vi "FTW-Messenger-AsynchronousInitRequest.vi"(0 "Messenger Type":refnum<class "FTW-Messenger.lvclass">, 11 "error in":errorcluster) -> (4 "Messenger":refnum<class "FTW-Messenger.lvclass">, 15 "error out":errorcluster)   [LabVIEW 2013, in "FTW-Messenger.lvclass"]
uses:
  FTW-Messenger.lvclass
  Container/FTW-Container.lvclass
  FTW-Messenger.lvclass/FTW-Messenger.ctl
panel:
  # "Inputs"
  # "Outputs"
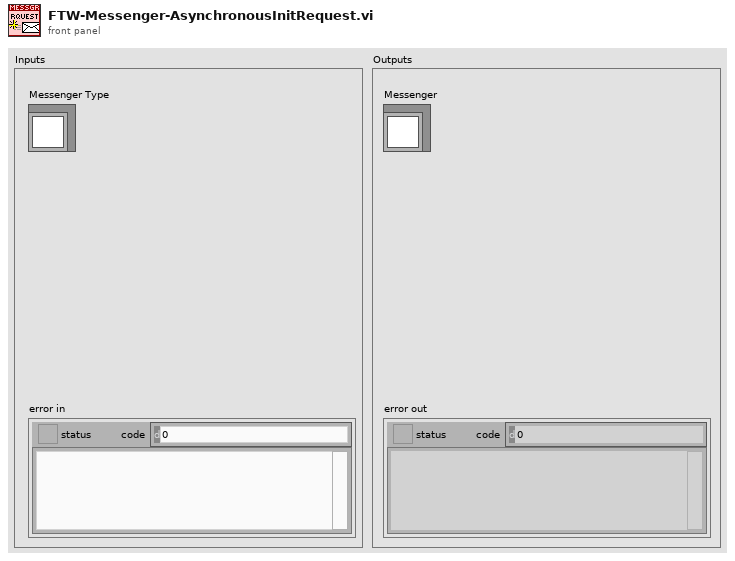
[diagram p1: front panel]
types:
  T1 = cluster{"Response":refnum<class "FTW-Container.lvclass">, "Messenger":refnum<class>}
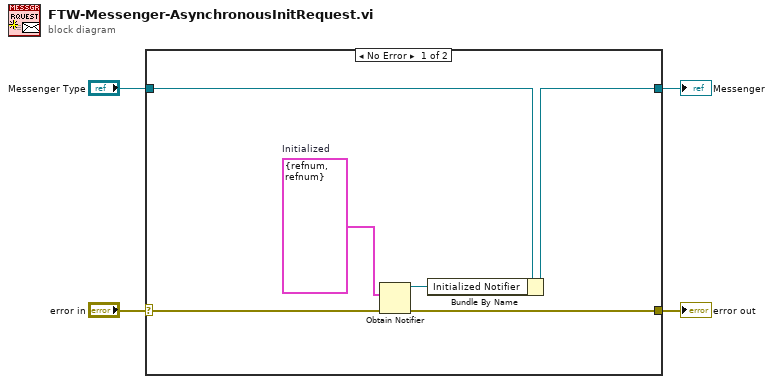
[diagram p0: block diagram]
diagram:
  n1 = case shown="No Error" "error in" {
    selector: "error in" -> [w10 w12]
    tunnel: [w8 w12] -> w3
    tunnel: [w9 w11] -> w4
    tunnel: "Messenger Type" -> [w7 w11]
    frame No Error {
      w5 = T1 {"Response"=refnum, "Messenger"=refnum}  # Initialized
      n2 = Obtain Notifier(notification data type=w5, error in (no error)=w10) -> (notifier out=w6:refnum<notifier>, error out=w8:errorcluster)  [unwired: 2 in, 1 out]
      n3 = Bundle By Name(cluster=w7, "Initialized Notifier"=w6) -> (w9:refnum<class "FTW-Messenger.lvclass">)
    }
    frame Error {
    }
  }
  "Messenger" <- w4
  "error out" <- w3
